vi "calcDifferenceFromAmbient.vi"(8 "error in (no error)":errorcluster, 11 "Thermocouple in":refnum<class "Thermocouple.lvclass">) -> (0 "error out":errorcluster, 3 "Thermocouple out":refnum<class "Thermocouple.lvclass">)   [LabVIEW 2013, in "Thermocouple.lvclass"]
uses:
  Thermocouple.lvclass
  Thermocouple.lvclass/Thermocouple.ctl
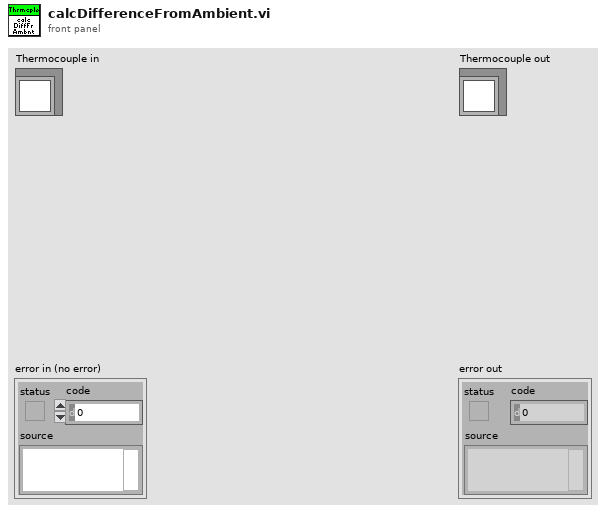
[diagram p1: front panel]
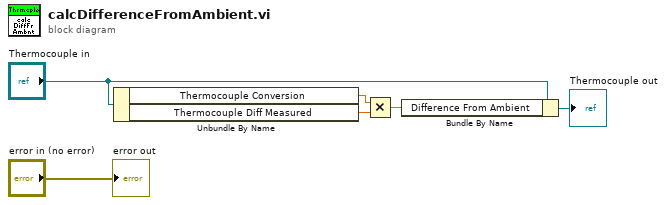
[diagram p0: block diagram]
diagram:
  n1 = Unbundle By Name("Thermocouple in") -> ("Thermocouple Conversion"=w5:dbl[unit], "Thermocouple Diff Measured"=w2:dbl[unit])
  n2 = Multiply(x=w5, y=w2) -> (x*y=w1:dbl[unit])
  n3 = Bundle By Name(cluster="Thermocouple in", "Difference From Ambient"=w1) -> (→"Thermocouple out":refnum<class "Thermocouple.lvclass">)
  "error out" <- "error in (no error)"
